vi "P 4 Convert Units.vi"(9 "P 4":T1 {"Default stroker force limit (tonne)" format="%.2f"; "Stroker Relay 2" format="%.2f"; "Stroker relay 1" format="%.2f"; "Tacometer puls" format="%.2f"; "Anchor Enabled Pressure" format="%.2f"; "Stroke force lim." format="%.2f"; "Stroker Solenoid limit" format="%.2f"}) -> (1 "P 4":T1 {"Default stroker force limit (tonne)" format="%.2f"; "Stroker Relay 2" format="%.2f"; "Stroker relay 1" format="%.2f"; "Tacometer puls" format="%.2f"; "Anchor Enabled Pressure" format="%.2f"; "Stroke force lim." format="%.2f"; "Stroker Solenoid limit" format="%.2f"}, 5 "Unit":string)   [LabVIEW 2011]
uses:
  Options Page 4.ctl
  Tool/Stroke force selector.ctl
  Tool/Default anchor behavior.ctl
  Tool/Default stroker behavior.ctl
  GUI/Controls/Slips Type Radio.ctl
  Tool/Variable List Tool Analog.ctl
panel:
  # "ms"
  # "When both relays are used in \nthe same operation, the lowest\nlimit is used for both."
  # "A"
  # "A"
  # "A"
  # "Bar"
  # "ms"
  # "When both relays are used in \nthe same operation, the lowest\nlimit is used for both."
  # "A"
  # "A"
  # "A"
  # "Bar"
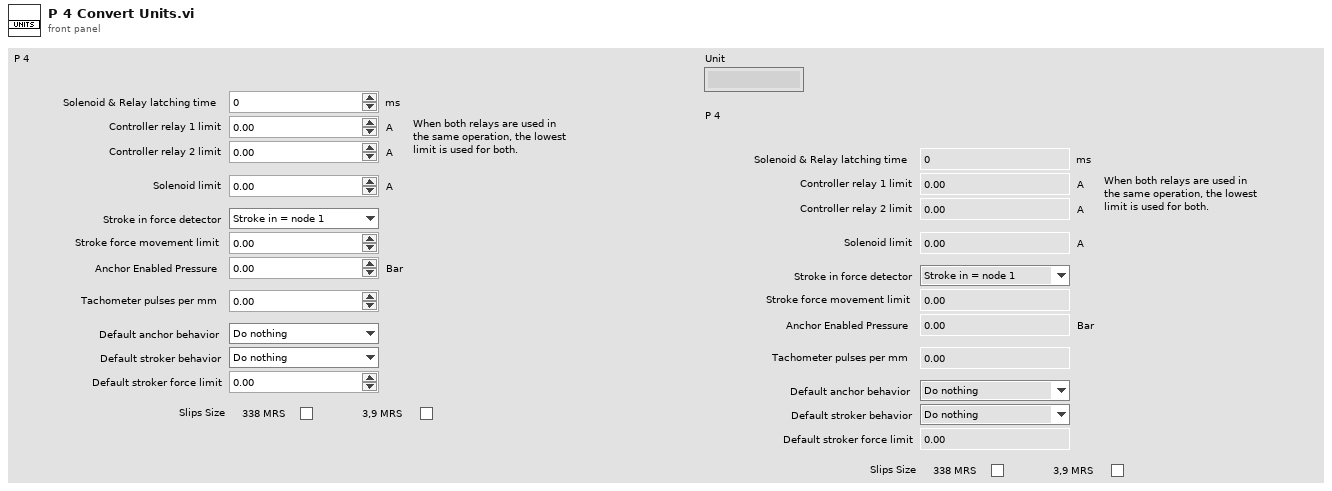
[diagram p1: front panel]
types:
  T1 = typedef "Options Page 4.ctl" = cluster{"Solenoid & Relay latching time":u16, "Stroker relay 1":dbl, "Stroker Relay 2":dbl, "Stroker Solenoid limit":dbl, "Force det.":T2, "Stroke force lim.":dbl, "Anchor Enabled Pressure":dbl, "Tacometer puls":dbl, "Default anchor behavior":T3, "Default stroker behavior":T4, "Default stroker force limit (tonne)":dbl, "Slips Size":T5}
  T2 = typedef "Stroke force selector.ctl" = enum16{"Stroke in = node 1", "Strok out = node 1"}
  T3 = typedef "Default anchor behavior.ctl" = enum16{"Do nothing", "Set Anchor", "Release Anchor"}
  T4 = typedef "Default stroker behavior.ctl" = enum16{"Do nothing", "Stop", "Go Out", "Go In"}
  T5 = typedef "Slips Type Radio.ctl" = enum32{"No Selection", "338 MRS", "3,9 MRS"}
  T6 = typedef "Variable List Tool Analog.ctl" = enum16{"Tool Max Temperature", "Tool (Controller) Temperature", "Tool Supply Voltage", "Tool (Controller) Current", "Tool Acceleration X", "Tool Acceleration Y", "Tool Acceleration Z", "Tool Acceleration Sum", "Tool Inclination", "Tool Rotation", "Tool GP Sensor 1", "Tool GP Sensor 2", "Tool (Pressure 1) Temperature", "Tool Pressure 1 RAW", "Tool (Pressure 2) Temperature", "Tool Pressure 2 RAW", "Tool (Solenoid) Temperature", "Tool Solenoid Position", "PSU Temp", "Head Voltage", "PSU Main Voltage out", "PSU Main Current out", "Upper Tension Sub Temp", "Tool Upper Tension Sub Raw", "Lower Tension Sub Temp", "Tool Lower Tension Sub Raw", "Tool Var27 - Reserved", "Tool Var28 - Reserved", "Tool Var29 - Reserved", "Tool Var30 - Reserved", "Stroke Extension", "Stroke In Force", "Stroke Out Force", "Stroke Force", "Stroker Pressure 1", "Stroker Pressure 2", "Stroker Upper Tension Sub", "Stroker Lower Tension Sub", "Stroker Var09 - Reserved", "Stroker Var10 - Reserved", "Tractor Upper Tension Sub", "Tractor Lower Tension Sub", "Tractor Var03 - Reserved", "Tractor Var04 - Reserved", "Tool Temperature sensor", "Tool Motor Voltage", "Tool Motor Current", "Tool Motor Torque", "Tool weight on bit", "Tool Motor RPM"}
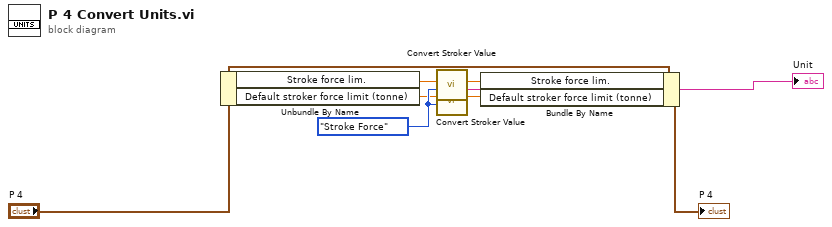
[diagram p0: block diagram]
diagram:
  w8 = Variable_List_Tool_Analog."Stroke Force" ("Variable ID")
  n1 = Unbundle By Name("P 4") -> ("Stroke force lim."=w2:dbl, "Default stroker force limit (tonne)"=w4:dbl)
  n2 = call "Convert Stroker Value.vi"("Variable"=w8, "Value in"=w2) -> ("Unit"=→"Unit":string, "Converted value"=w3:dbl)  [unwired: 8 in]
  n3 = call "Convert Stroker Value.vi"("Variable"=w8, "Value in"=w4) -> ("Converted value"=w5:dbl)  [unwired: 8 in, 1 out]
  n4 = Bundle By Name(cluster="P 4", "Stroke force lim."=w3, "Default stroker force limit (tonne)"=w5) -> (→"P 4":T1)
